vi "configure.vi"(8 "error in (no error)":errorcluster, 11 "Hardware in":refnum<class "Hardware.lvclass">) -> (0 "error out":errorcluster, 3 "Hardware out":refnum<class "Hardware.lvclass">)   [LabVIEW 2026, in "Hardware.lvlib" / "Hardware.lvclass"]
uses:
  Hardware.lvclass
  Hardware.lvclass/Hardware.ctl
  HW Config/HW Configuration.lvclass/HW Configuration.ctl
  HW Config/Read IO Mapping.vi
  HW Config/HW Configuration.lvclass
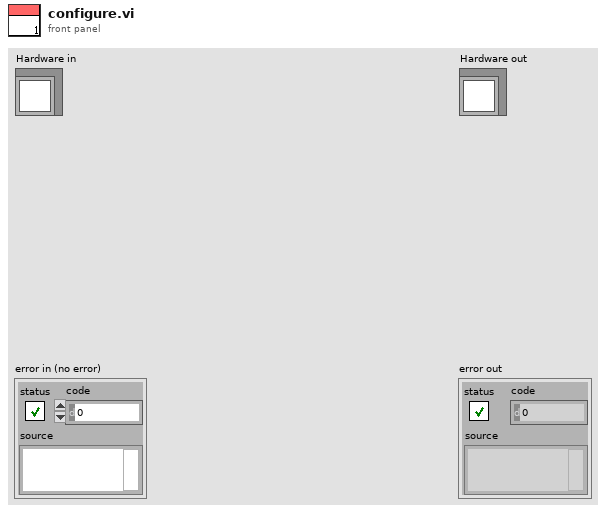
[diagram p1: front panel]
types:
  T1 = cluster{"Device Name":string, "Channel Mapping (Device -> Channel)":string[][]}
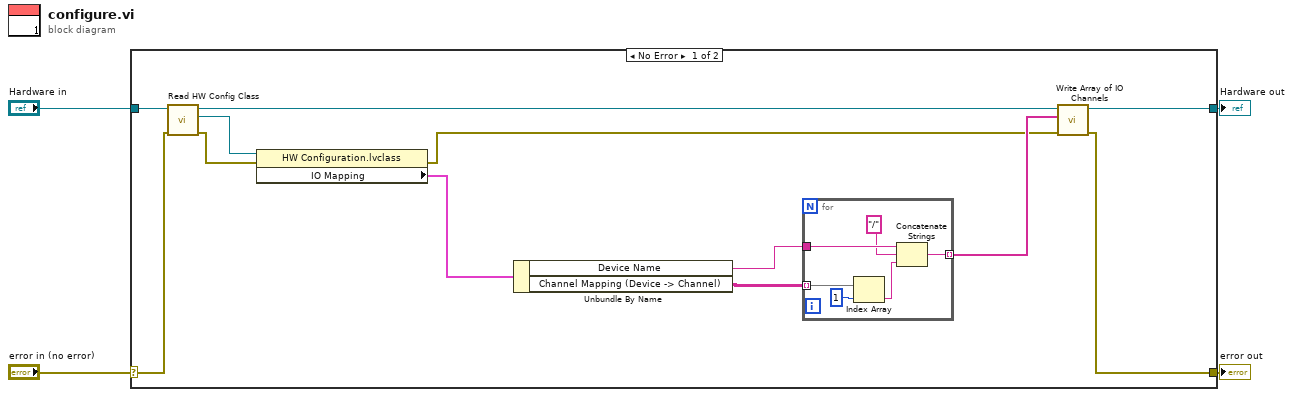
[diagram p0: block diagram]
diagram:
  n1 = case shown="No Error" "error in (no error)" {
    selector: "error in (no error)" -> [w9 w24]
    tunnel: [w10 w24] -> w3
    tunnel: [w11 w23] -> w1
    tunnel: "Hardware in" -> [w8 w23]
    frame No Error {
      n2 = call "Read HW Config Class.vi"("error in (no error)"=w9, "Hardware in"=w8) -> ("error out"=w6:errorcluster, "Hardware.lvlib:HW Configuration.lvclass"=w16:refnum<class "HW Configuration.lvclass">, "Hardware out"=w7:refnum<class "Hardware.lvclass">)  [unwired: 7 in]
      n3 = property class="HW Configuration.lvclass"(reference=w16, error in=w6) -> (error out=w5:errorcluster, "IO Mapping"=w15:T1)  [unwired: 1 out]
      n4 = Unbundle By Name(w15) -> ("Device Name"=w13:string, "Channel Mapping (Device -> Channel)"=w14:string[][])
      n5 = for {
        tunnel: w14 -> [w22] mode=indexing
        tunnel: [w19] -> w12 mode=indexing
        tunnel: w13 -> [w18]
        n6 = Index Array(array=w22, index=1) -> (element=w20:string)
        n7 = Concatenate Strings(w18, "/" ("string"), w20) -> (w19:string)
      }
      n8 = call "Write Array of IO Channels.vi"("error in (no error)"=w5, "Array of IO Channels"=w12, "Hardware in"=w7) -> ("error out"=w10:errorcluster, "Hardware out"=w11:refnum<class "Hardware.lvclass">)  [unwired: 7 in]
    }
    frame Error {
    }
  }
  "error out" <- w3
  "Hardware out" <- w1
